vi "weight_old.vi"(10 "Q3":dbl caption="mg/s" format="%#.0f", 11 "PV weight":dbl caption="g" format="%#.0f") -> (2 "Q 1":dbl caption="mg/s" format="%#.0f", 3 "Weight 1":dbl caption="g" format="%#.0f", 5 "This VI":refnum<vi>)   [LabVIEW 2019]
panel:
  in  "Tab Control":T1(tab)
  out "dM 3":dbl caption="g" format="%#.0f"
  out "dM 1":dbl caption="g" format="%#.0f"
  in  "Tare":dbl caption="g" format="%#.0f"
  in  "<0>":bool
  in  "<вес>":bool
  out "k":dbl caption="g" format="%#.3f"
  in  "Вес":dbl caption="g" format="%#.0f"
  # "Усреднение за 1 мин"
  # "(расход)"
  # "Усреднение за 3 мин"
  # "(расход)"
  # "Вес тары (запомнить Weight 1)"
  # "Вес тары (ввести фактический вес-тара)"
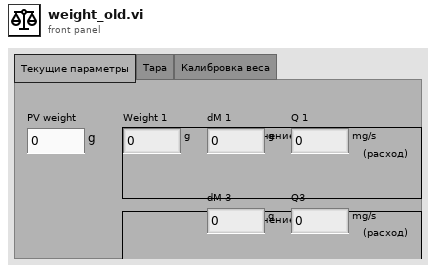
[diagram p1: front panel]
types:
  T1 = enum32{"Текущие параметры", "Тара", "Калибровка веса"}
  T2 = typedef "AI_gm3.ctl" = enum16{"EB31_BJ1", "EB31BA1_XQ01", "EB31BC2_XQ01", "EB31BT1_XQ01", "EB31BT3_XQ01", "EB321_BE1", "EB321_BJ1", "EB321BA1_XQ01", "EB321BC2_XQ01", "EB321BT1_XQ01", "EB322_BE1", "EB322_BJ1", "EB322BA1_XQ01", "EB322BC2_XQ01", "EB322BT1_XQ01", "EB323_BE1", "EB323_BJ1", "EB323BA1_XQ01", "EB323BC2_XQ01", "EB323BT1_XQ01", "EB32BT3_XQ01", "EB3BP1_XQ01", "EB3QN1_XQ01", "EB3QN2_XQ01", "GM31BP1_XQ01", "GM31BW1_XQ01", "GM31BW1_XZ01", "GM31BW1_BQ01", "GM31BW1_BQ03", "GM31QN1_XQ01", "GM32BP1_XQ01", "GM32QN1_XQ01", "GM32QN2_XQ01", "GM3HT1BC1_XQ01", "GM3HT1BT1_XQ01", "GM3HT1BC2_XQ01", "GM3HT1BT2_XQ01", "GM2EP1BT1_XQ01", "GM2EP1BT2_XQ01", "GM2EP1BT3_XQ01", "GM2EP1BT4_XQ01", "GM2EP1BT5_XQ01", "GM2EP1BT6_XQ01", "GM2EP1BT7_XQ01", "GM2EP1BT8_XQ01", "GM2EP1BT9_XQ01", "GM31BP2_XQ01"}
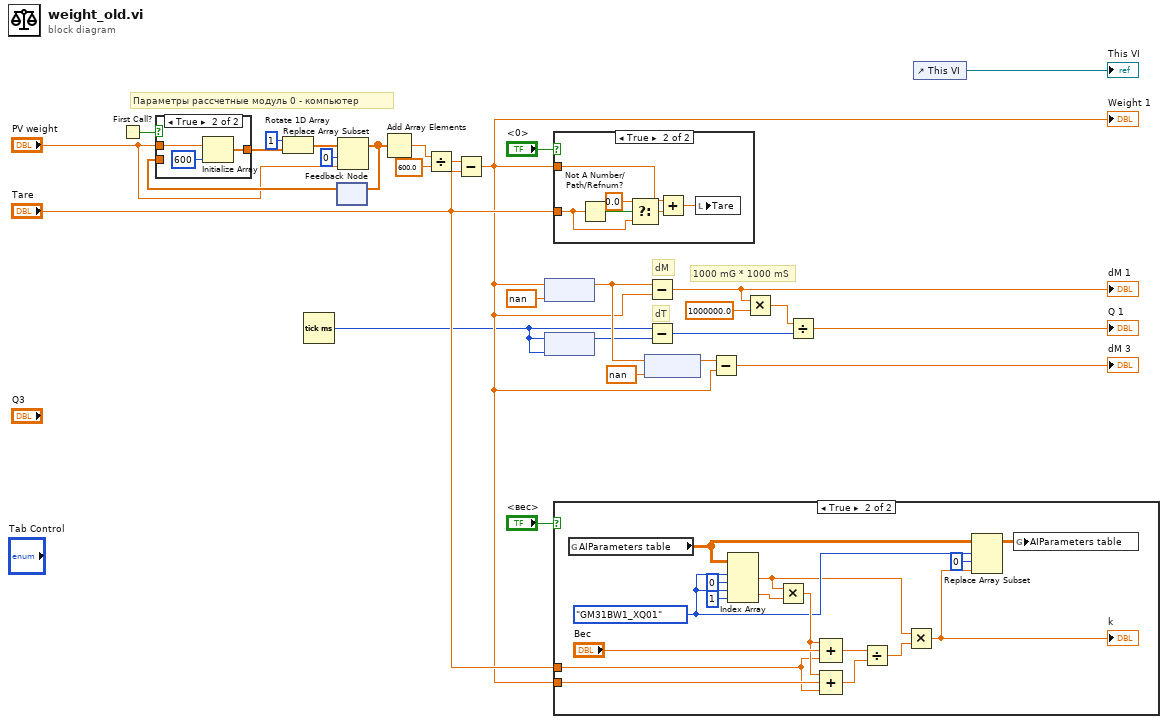
[diagram p0: block diagram]
diagram:
  # "1000 mG * 1000 mS"
  # "dM"
  # "dT"
  # "Параметры рассчетные модуль 0 - компьютер"
  n1 = First Call?() -> (First Call?: T/F=w19:bool)
  n2 = Tick Count (ms)() -> (millisecond timer value=w7:u32)
  n3 = feedback #1() -> (w21:dbl[])  [unwired: 1 in]
  n4 = case shown="True" w19 {
    tunnel: [w29 w31] -> w20
    tunnel: "PV weight" -> [_ w30]
    tunnel: w21 -> [w29 _]
    frame False {
    }
    frame True {
      n5 = Initialize Array(w30, 600 ("dimension size")) -> (w31:dbl[])
    }
  }
  n6 = Rotate 1D Array(1:w20, 2:1 ("n")) -> (0:w27:dbl[])
  n7 = Replace Array Subset(array=w27, new element="PV weight", index=0) -> (w25:dbl[])
  n8 = feedback-in #1(w25) -> ()
  n9 = Add Array Elements(numeric array=w25) -> (sum=w23:dbl)
  n10 = Divide(x=w23, y=600.0) -> (x/y=w22:dbl)
  n11 = Subtract(x=w22, y="Tare") -> (x-y=w9:dbl)
  "Weight 1" <- w9
  n12 = feedback #2(nan) -> (w14:dbl)
  n13 = feedback-in #2(w9) -> ()
  n14 = feedback #3(w7) -> (w6:u32)
  n15 = feedback-in #3(w7) -> ()
  n16 = case shown="True" "<0>" {
    tunnel: "Tare" -> [_ w36]
    tunnel: w9 -> [_ w34]
    frame False {
    }
    frame True {
      n17 = Not A Number/Path/Refnum?(number/path/refnum=w36) -> (NaN/Path/Refnum?=w38:bool)
      n18 = Select(t=0.0 ("y"), s=w38, f=w36) -> (s? t:f=w33:dbl)
      n19 = Add(x=w34, y=w33) -> (x+y=w35:dbl)
      n20 = local write "Tare"(w35) -> ()
    }
  }
  n21 = case shown="True" "<вес>" {
    tunnel: w9 -> [_ w50]
    tunnel: "Tare" -> [_ w42]
    frame False {
    }
    frame True {
      w45 = AI_gm3."GM31BW1_XQ01" ("AI 2")
      n22 = global read "h_gm1_parameters_181001.vi" "AIParameters table"() -> (w46:dbl[][])
      n23 = Index Array(array=w46, index (row) #1=w45, index (col) #1=0 ("disabled index (col)"), index (row) #2=w45, index (col) #2=1 ("disabled index (col)")) -> (element #1=w41:dbl, element #2=w52:dbl)
      n24 = Multiply(x=w41, y=w52) -> (x*y=w47:dbl)
      n25 = Compound Arithmetic op=ADD(w47, "Вес", w42) -> (w49:dbl)
      n26 = Compound Arithmetic op=ADD(w47, w50, w42) -> (w48:dbl)
      n27 = Divide(x=w49, y=w48) -> (x/y=w39:dbl)
      n28 = Multiply(x=w41, y=w39) -> (x*y=w40:dbl)
      "k" <- w40
      n29 = Replace Array Subset(array=w46, new element=w40, index (row)=w45, index (col)=0 ("disabled index (col)")) -> (w43:dbl[][])
      n30 = global write "h_gm1_parameters_181001.vi" "AIParameters table"(w43) -> ()
    }
  }
  n31 = feedback #4(nan) -> (w15:dbl)
  n32 = feedback-in #4(w14) -> ()
  n33 = Subtract(x=w14, y=w9) -> (x-y=w4:dbl)
  "dM 1" <- w4
  n34 = Subtract(x=w7, y=w6) -> (x-y=w2:u32)
  n35 = Subtract(x=w15, y=w9) -> (x-y=→"dM 3":dbl)
  n36 = Multiply(x=w4, y=1000000.0) -> (x*y=w3:dbl)
  n37 = Divide(x=w3, y=w2) -> (x/y=→"Q 1":dbl)
  n38 = control-ref of="This VI"() -> (→"This VI":refnum<vi>)
